vi "Close.vi"(8 "error in (no error)":errorcluster, 11 "FormulaLV App in":refnum<class "FormulaG App.lvclass">) -> (0 "error out":errorcluster)   [LabVIEW 2020, in "FormulaG.lvlib" / "FormulaG App.lvclass"]
uses:
  FormulaG App.lvclass
  FormulaG App.lvclass/FormulaG App.ctl
  <vilib>/IlluminatedG/IG HTTP Server/HTTP Server/Server/Server.lvclass
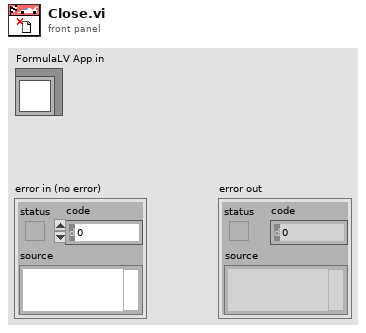
[diagram p1: front panel]
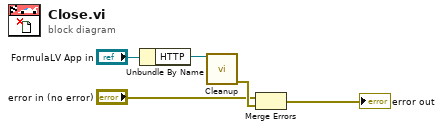
[diagram p0: block diagram]
diagram:
  n1 = Unbundle By Name("FormulaLV App in") -> ("HTTP"=w4:refnum<class "Server.lvclass">)
  n2 = call <vilib>:"Cleanup.vi"("Server in"=w4) -> ("error out"=w3:errorcluster)  [unwired: 10 in]
  n3 = Merge Errors("error in (no error)", w3) -> (→"error out":errorcluster)
